vi "Test Uart.vi"() -> ()   [LabVIEW 2014]
uses:
  <vilib>/Instr/_visa.llb/VISA Open Access Mode.ctl
  <vilib>/MakerHub/LINX/Public/Peripherals/UART/UART Write String.vi
  <vilib>/MakerHub/LINX/Public/Peripherals/UART/UART Write Byte Array.vi
  <vilib>/MakerHub/LINX/Private/Local IO/LinxUartWrite.vi
  <vilib>/MakerHub/LINX/Public/Utilities/Check Channel.vi
  <vilib>/MakerHub/LINX/Private/Local IO/Handle Errors.vi
  <vilib>/MakerHub/LINX/Public/Utilities/Open Local.vi
  <vilib>/MakerHub/LINX/Private/Utilties/Generate Error.vi
  <vilib>/MakerHub/LINX/Public/Peripherals/UART/UART Read String.vi
  <vilib>/MakerHub/LINX/LMH-LINX.lvlib
panel:
  out "read buffer":string
  out "Error Out":errorcluster
  out "Data":string
  out "find list":string[](array[string])
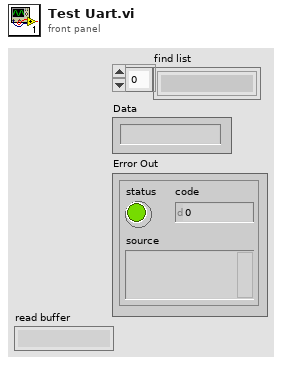
[diagram p1: front panel]
types:
  T1 = typedef "VISA Open Access Mode.ctl" = u32
  T2 = typedef "LMH-LINX.lvlib/LINX Ref.ctl" = cluster{"IO":T3, "Interface":T4, "LINX Device Config":T5}
  T3 = typedef "LMH-LINX.lvlib/Platform.ctl" = enum16{"Remote", "Local"}
  T4 = typedef "LMH-LINX.lvlib/Interface.ctl" = enum16{"Serial", "TCP"}
  T5 = typedef "LMH-LINX.lvlib/Device.lvlib/LINX Device Config.ctl" = cluster{"Interface":T4, "COM Port":refnum<visa-resource-name>, "TCP Configuration":T6, "Device Family":u8, "Device ID":u8, "Device Name":string, "TCP Ref":refnum<k5>, "Channels":T7}
  T6 = typedef "LMH-LINX.lvlib/Device.lvlib/TCP Config.ctl" = cluster{"IP Address":string, "Port":u16}
  T7 = typedef "LMH-LINX.lvlib/Channels.ctl" = cluster{"DI":u8[], "DO":u8[], "AI":u8[], "AO":u8[], "PWM":u8[], "QE":u8[], "UART":u8[], "I2C 2":u8[], "SPI":u8[], "CAN":u8[], "Servo":u8[], "AI Ref (V)":dbl, "AI Resolution (Bits)":u8, "AO Ref (V)":dbl, "AO Resolution (Bits)":u8}
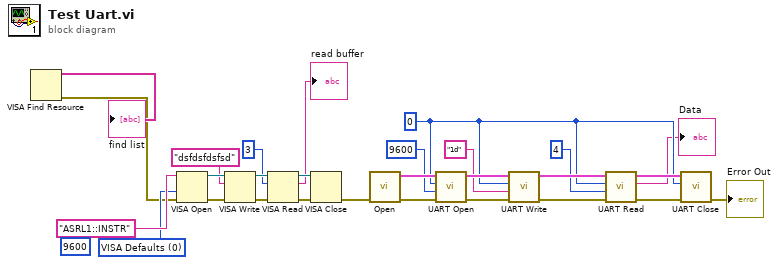
[diagram p0: block diagram]
diagram:
  w12 = T1 0 items=["VISA Defaults"=0, "Exclusive Lock"=1, "Load Configured Settings"=4] ("Access Mode")
  w16 = u8 0 ("UART Channel (0)")
  (unwired) u32 9600 ("Baud Rate Override")
  n1 = VISA Find Resource() -> (0:w11:errorcluster, 3:→"find list":string[])  [unwired: 3 in, 1 out]
  n2 = VISA Open(access mode=w12, error in (no error)=w11, VISA resource name="ASRL1::INSTR") -> (VISA resource name=w10:refnum<visa-resource-name>, error out=w9:errorcluster)  [unwired: 2 in]
  n3 = VISA Write(VISA resource name=w10, write buffer="dsfdsfdsfsd", error in (no error)=w9) -> (VISA resource name out=w7:refnum<visa-resource-name>, error out=w6:errorcluster)  [unwired: 1 out]
  n4 = VISA Read(VISA resource name=w7, byte count=u32 3, error in (no error)=w6) -> (VISA resource name out=w4:refnum<visa-resource-name>, read buffer=→"read buffer":string, error out=w3:errorcluster)  [unwired: 1 out]
  n5 = VISA Close(VISA resource name=w4, error in (no error)=w3) -> (error out=w1:errorcluster)
  n6 = call-poly <vilib>:"Open.vi"("Error In"=w1) -> ("Error Out"=w26:errorcluster, "LINX Resource"=w27:T2)  [unwired: 8 in, 1 out]
  n7 = call <vilib>:"UART Open.vi"("Error In"=w26, "Baud Rate (9600)"=u32 9600, "UART Channel (0)"=w16, "LINX Resource"=w27) -> ("Error Out"=w22:errorcluster, "LINX Resource"=w24:T2)  [unwired: 5 in, 1 out]
  n8 = call-poly <vilib>:"UART Write.vi"("Error In"=w22, "Data"="1d", "UART Channel (0)"=w16, "LINX Resource"=w24) -> ("Error Out"=w21:errorcluster, "LINX Resource"=w23:T2)  [unwired: 6 in]
  n9 = call-poly <vilib>:"UART Read.vi"("Error In"=w21, "Num Bytes"=u8 4, "UART Channel (0)"=w16, "LINX Resource"=w23) -> ("Error Out"=w17:errorcluster, "Data"=→"Data":string, "LINX Resource"=w18:T2)  [unwired: 5 in]
  n10 = call <vilib>:"UART Close.vi"("Error In"=w17, "UART Channel (0)"=w16, "LINX Resource"=w18) -> ("Error Out"=→"Error Out":errorcluster)  [unwired: 7 in, 1 out]
